vi "Main.vi"() -> ()   [LabVIEW 2013]
doc: "This template is for the Queued Message Handler design pattern.\n\nThe Event Handling Loop generates messages based on user interface actions.\n\nThe Message Handling Loop processes messages generated by the Event Handling Loop, or by other messages. The messages are string values, so new messages can be added easily to the Message Cases case structure in the Message Handling Loop. Each message cluster can also provide an optional value for Message Data, which is a variant that can be converted to whatever message-specific data is required."
uses:
  controls/UI Data.ctl
  Message Queue/Message Queue.lvlib
  User Event - Stop/User Event - Stop.lvlib
  <vilib>/vision/Image Controls.llb/IMAQ Image.ctl
  FPGA/FPGA Frame Grabbing.lvlib
  <vilib>/vision/NI_Vision_Development_Module.lvlib
  Image Processing/Image Processing.lvlib
  Common/State Machines/State Machine Lib.lvlib
  Message Passing/Main MsgQ.lvlib
  Message Passing/MsgQ Loops enum.ctl
  Sectors/Number of Wing Sector.ctl
panel:
  in  "Start Serial Server":bool=TRUE
  out "Wingbeat Amplitude Graph":dynamicdata(graph)
  in  "Stop Charts":bool
  in  "NumWingSectors":T1=12 items=["1"=1, "2"=2, "4"=4, "8"=8, "16"=16]
  in  "Wing ROIs":T2
  out "combo mask":T3(plugin-control)
  out "right \nannulus":T4={"Center X"=1090, "Center Y"=659, "Inner Radius"=200, "Outer Radius"=405, "Start Angle"=0.0, "End Angle"=90.0} {"End Angle" format="%.2f"; "Start Angle" format="%.2f"; "Center X" scale=0.0..1024.0}
  out "right masked image":T3(plugin-control)
  out "right mask":T3(plugin-control)
  out "left annulus":T4={"Center X"=929, "Center Y"=663, "Inner Radius"=200, "Outer Radius"=405, "Start Angle"=90.0, "End Angle"=180.0} {"End Angle" format="%.2f"; "Start Angle" format="%.2f"; "Center X" scale=0.0..1024.0}
  out "left masked image":T3(plugin-control)
  out "left mask":T3(plugin-control)
  in  "Accept Threshold":bool
  in  "Threshold Range":cluster{"Lower value":dbl, "Upper value":dbl}={"Lower value"=106.82432432432432, "Upper value"=255.0} {"Upper value" min=0.0 max=255.0 scale=0.0..255.0; "Lower value" min=0.0 max=255.0 scale=0.0..255.0}
  out "FPGA image info":T7={"Image Type"=0, "Unit"=enum."Undefined", "X Resolution"=2040, "Y Resolution"=1088, "X Step"=1.0, "Y Step"=1.0, "Image Name"="Image"} {"Image Type" items=["Grayscale (U8)", "Grayscale (I16)", "Grayscale (SGL)", "Complex (CSG)", "RGB (U32)", "HSL (U32)", "RGB (U64)", "Grayscale (U16)"]}
  out "Processed Image":T3(plugin-control)
  in  "Stream?":bool
  out "FPGA Image":T3(plugin-control)
  in  "Save Mask Coordinates":bool
  in  "Test Visual Response":bool
  in  "Test FPGA":bool
  out "Status Update":string="VI Stopped"
  in  "Define Mask":bool
  in  "Acquire Image":bool
  in  "Stop":bool
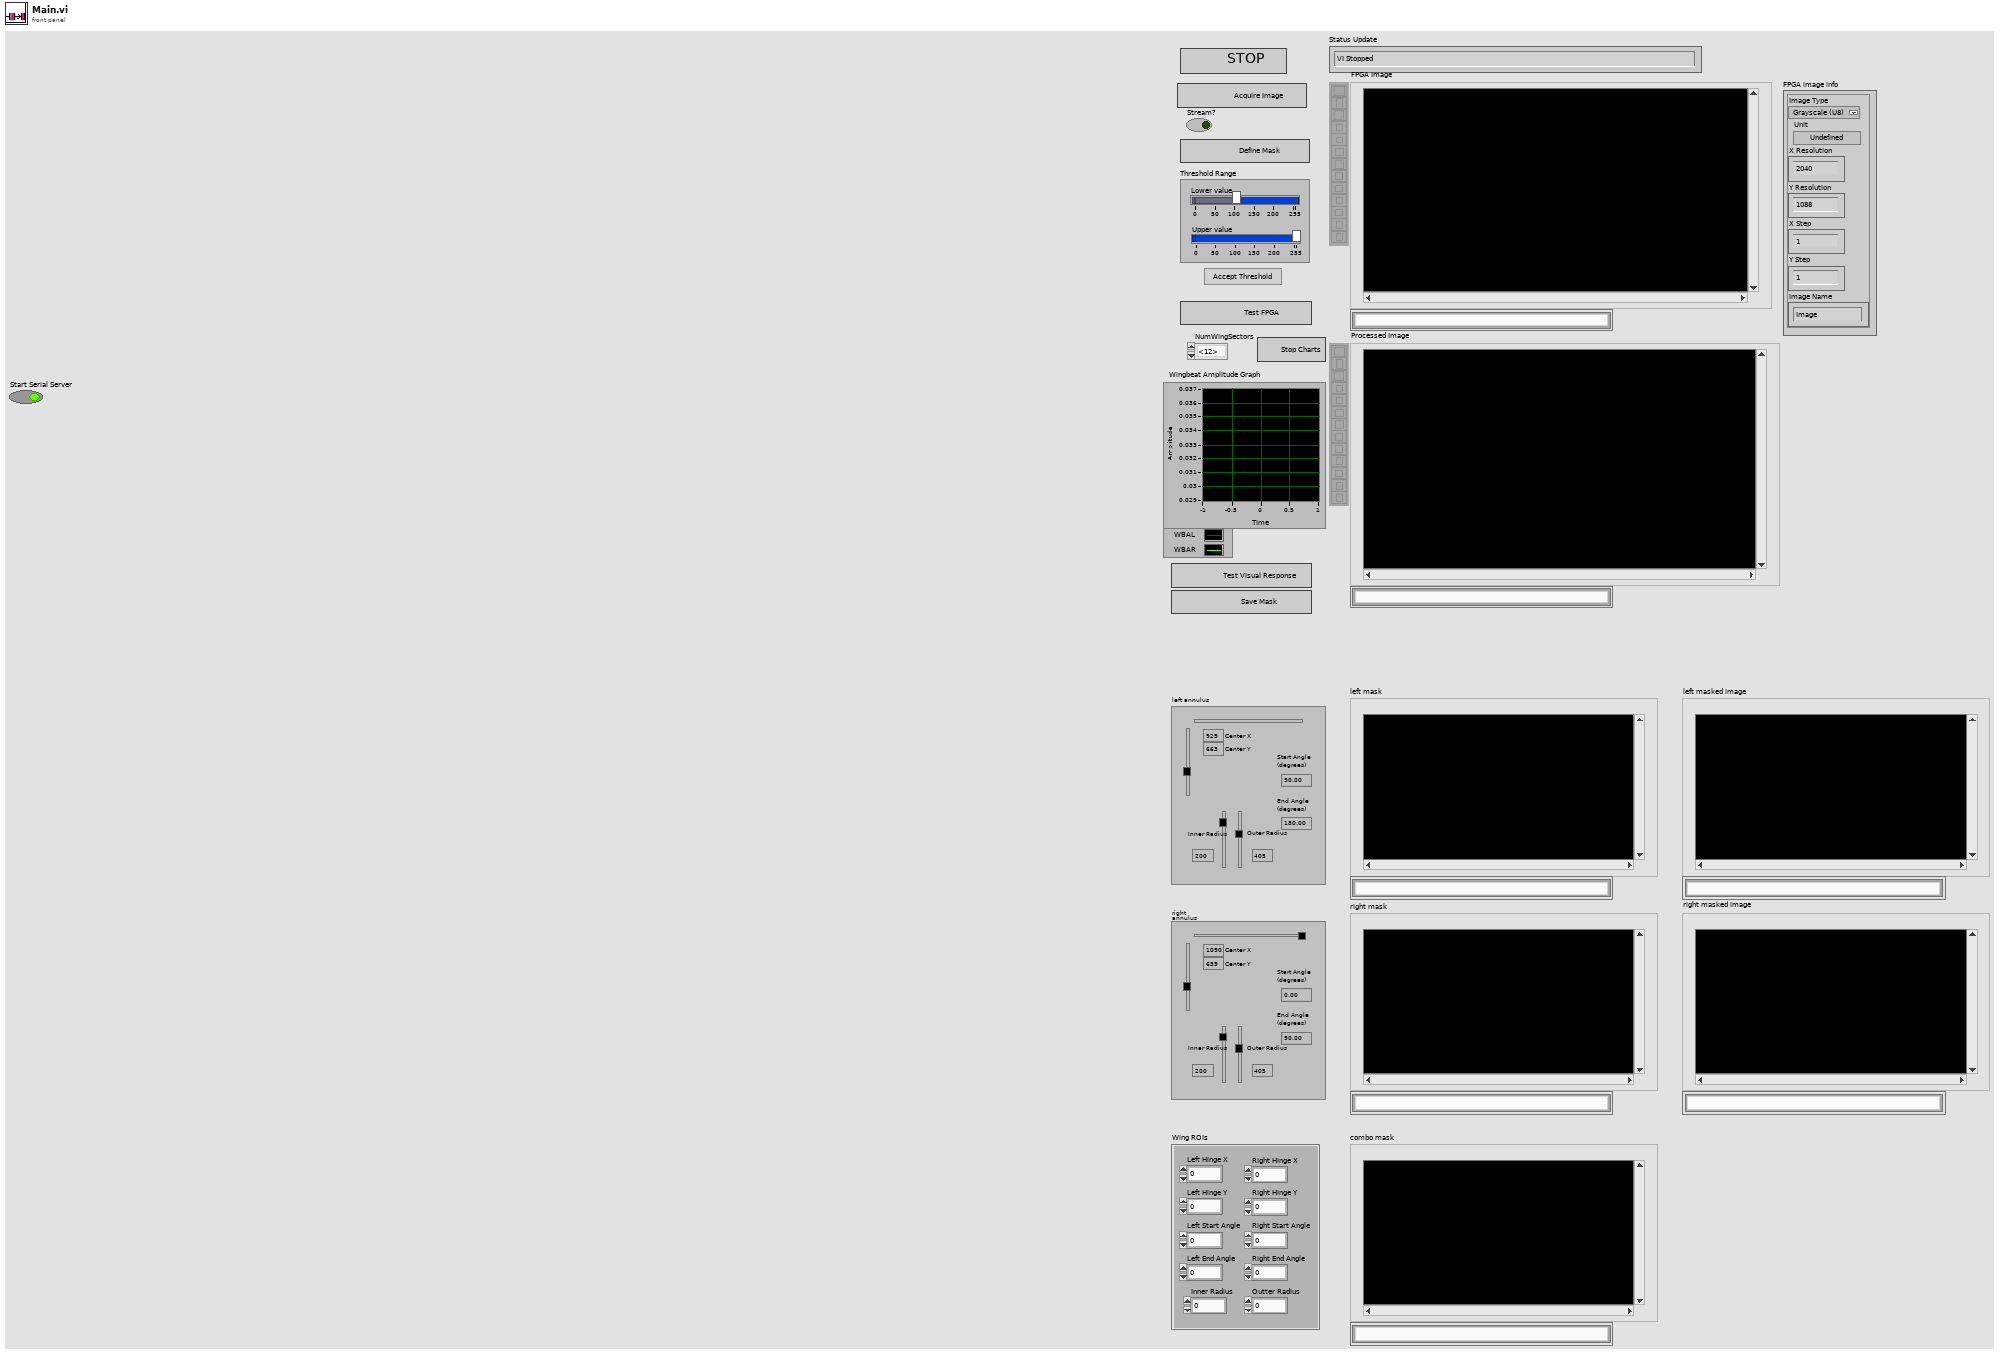
[diagram p1: front panel]
types:
  T1 = typedef "Number of Wing Sector.ctl" = u8
  T2 = cluster{"Left Hinge X":u16, "Left Hinge Y":u16, "Inner Radius":u16, "Outter Radius":u16, "Right Hinge X":u16, "Right Hinge Y":u16, "Right Start Angle":i16, "Right End Angle":i16, "Left Start Angle":i16, "Left End Angle":i16}
  T3 = typedef "IMAQ Image.ctl" = refnum<image>
  T4 = typedef "IMAQ Circle" = cluster{"Center X":i32, "Center Y":i32, "Inner Radius":i32, "Outer Radius":i32, "Start Angle":dbl, "End Angle":dbl}
  T5 = typedef "Image Type" = u32
  T6 = typedef "Image Unit" = enum32{"Undefined", "Angström", "Micrometer", "Millimeter", "Centimeter", "Meter", "Kilometer", "Microinch", "Inch", "Feet", "Nautical miles", "Standard miles", "Steps"}
  T7 = cluster{"Image Type":T5, "Unit":T6, "X Resolution":i32, "Y Resolution":i32, "X Step":sgl, "Y Step":sgl, "Image Name":string}
  T8 = typedef "UI Data.ctl" = cluster{"Boolean <Replace Me>":bool, "Initial Message":string, "Numeric <Replace Me>":dbl, "Acquire Image Ref":refnum<vi>, "Define Mask Ref":refnum<vi>, "Status Update Ref":refnum<vi>, "Stop Button Ref":refnum<vi>, "FPGA Image":T3, "Processed Image":T3, "Left Annulus":cluster{"Center X":i32, "Center Y":i32, "Inner Radius":i32, "Outer Radius":i32, "Start Angle":dbl, "End Angle":dbl}, "Right Annulus":cluster{"Center X":i32, "Center Y":i32, "Inner Radius":i32, "Outer Radius":i32, "Start Angle":dbl, "End Angle":dbl}}
  T9 = typedef "State Machine Lib.lvlib/STATE cluster.ctl" = cluster{"State":string, "Parameters":variant}
  T10 = typedef "Main MsgQ.lvlib/MsgQ Loops enum.ctl" = enum16{"User Interface", "Image Acq"}
  T11 = typedef "Message Queue.lvlib/All Message Queues.ctl" = cluster{"UI":refnum<queue>}
  T12 = cluster{"Center X":i32, "Center Y":i32, "Inner Radius":i32, "Outer Radius":i32, "Start Angle":dbl, "End Angle":dbl}
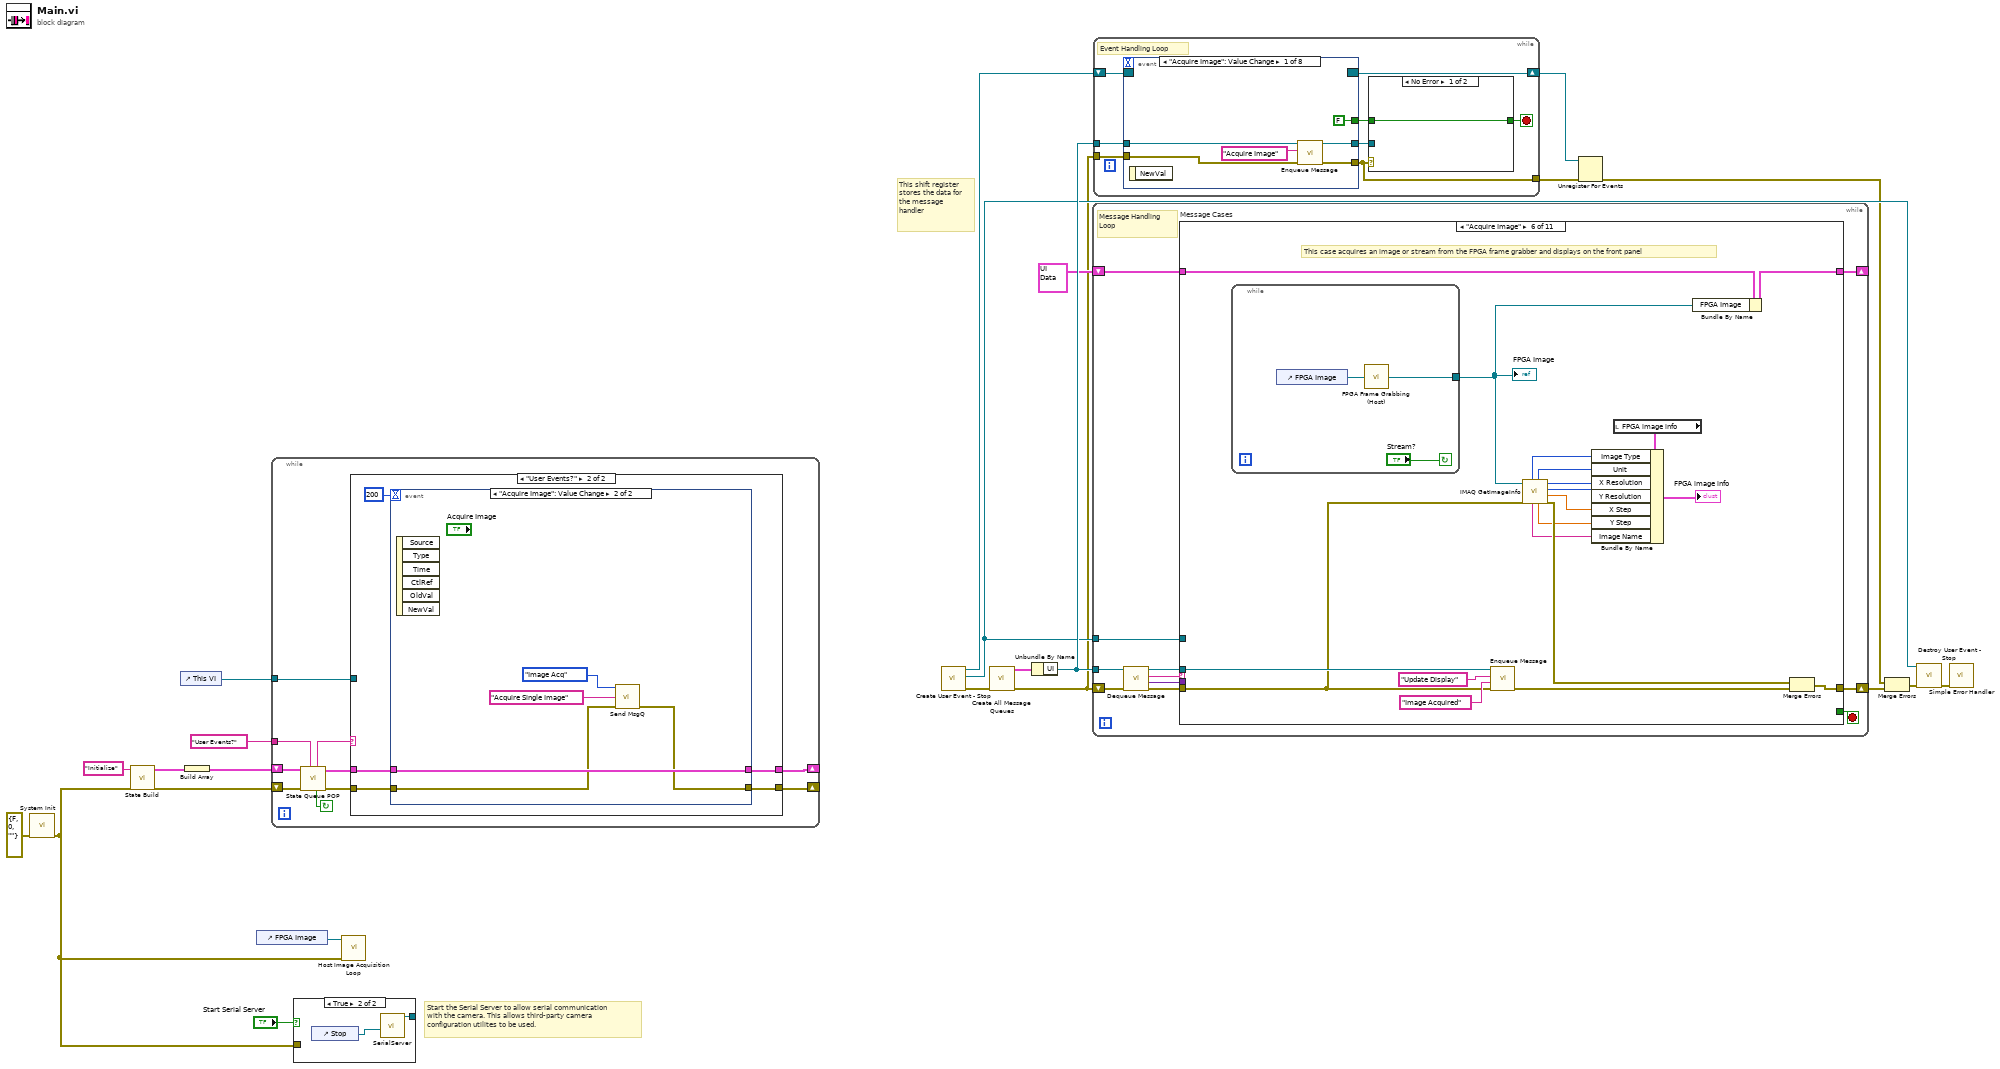
[diagram p0: block diagram]
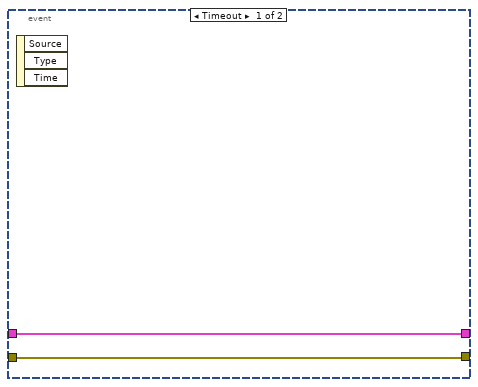
[diagram p3: hidden frame]
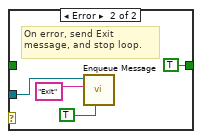
[diagram p5: hidden frame]
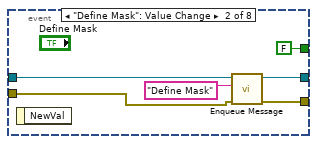
[diagram p6: hidden frame]
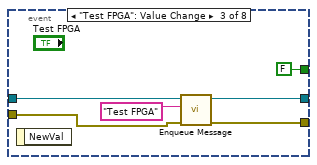
[diagram p7: hidden frame]
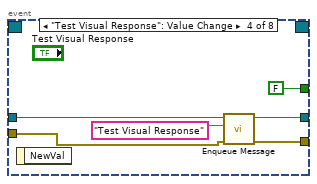
[diagram p8: hidden frame]
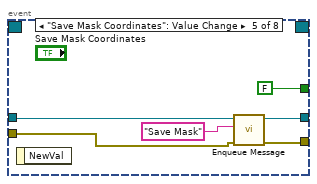
[diagram p9: hidden frame]
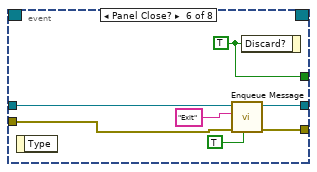
[diagram p10: hidden frame]
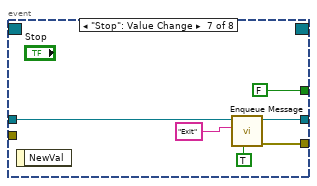
[diagram p11: hidden frame]
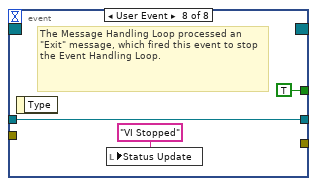
[diagram p12: hidden frame]
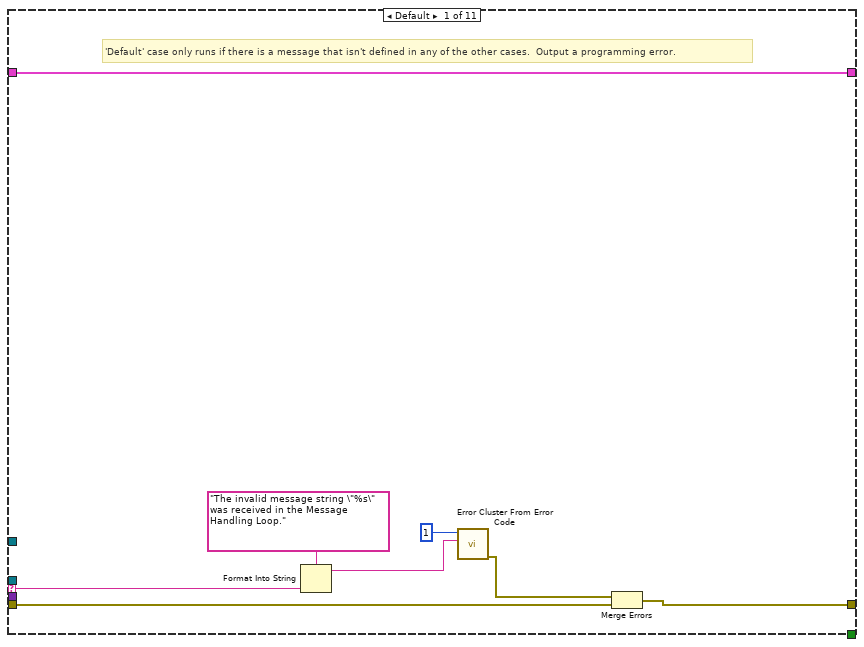
[diagram p13: hidden frame]
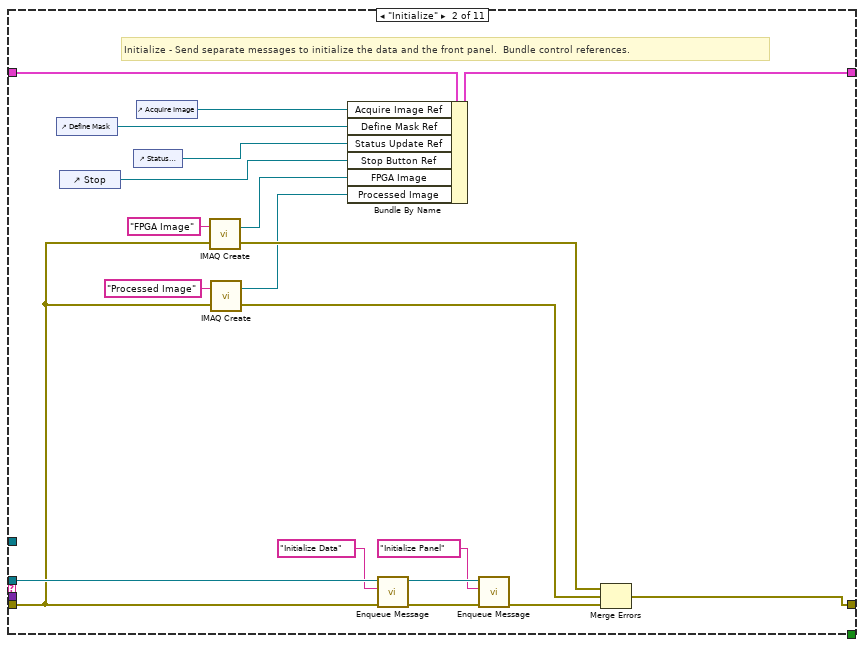
[diagram p14: hidden frame]
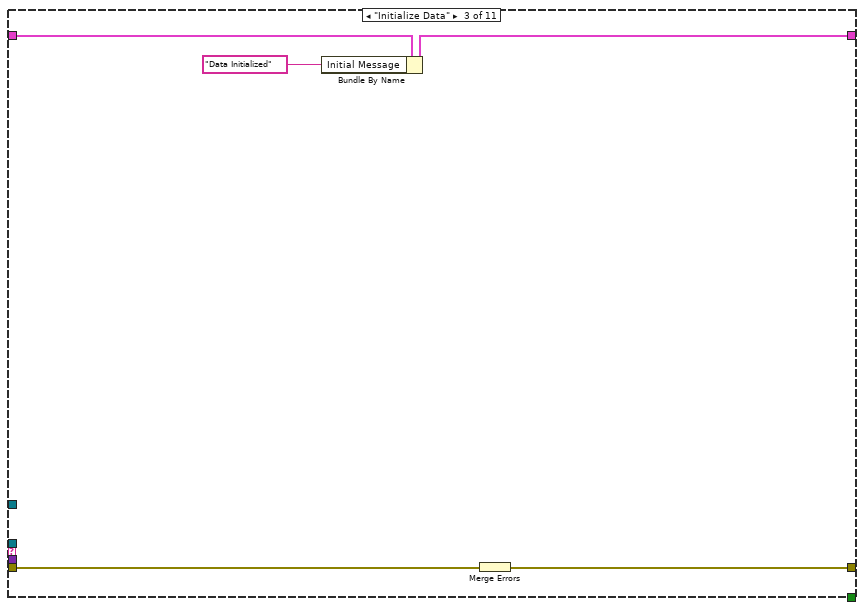
[diagram p15: hidden frame]
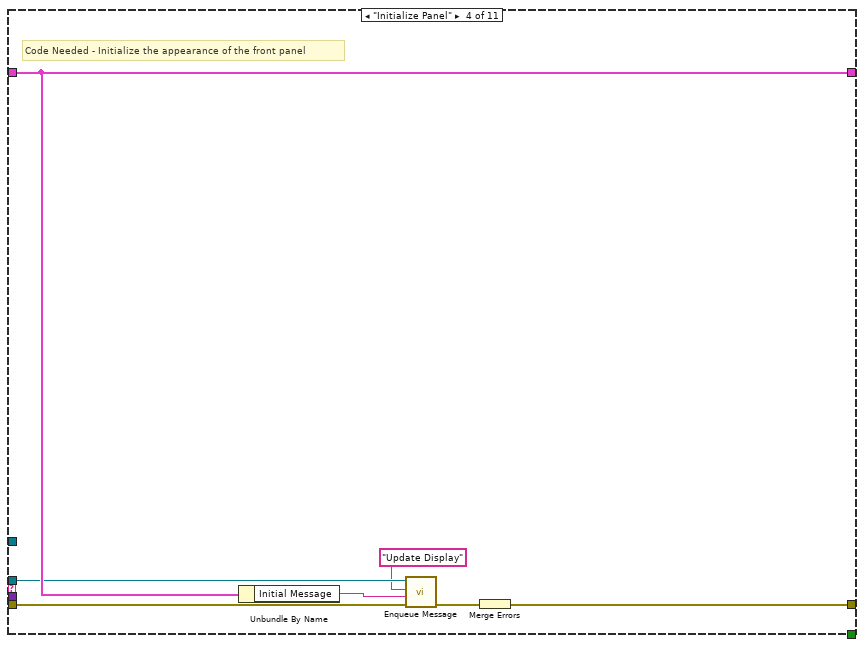
[diagram p16: hidden frame]
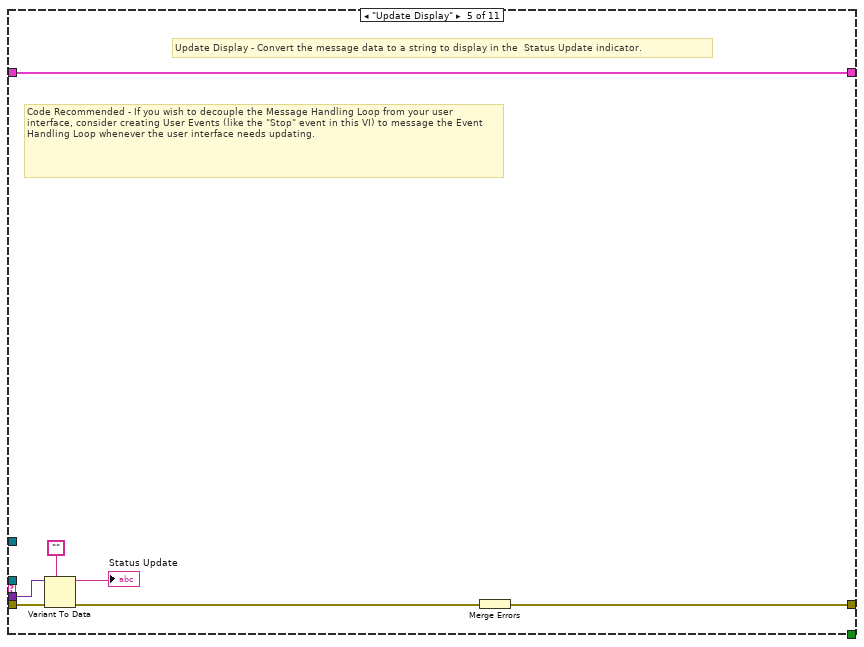
[diagram p17: hidden frame]
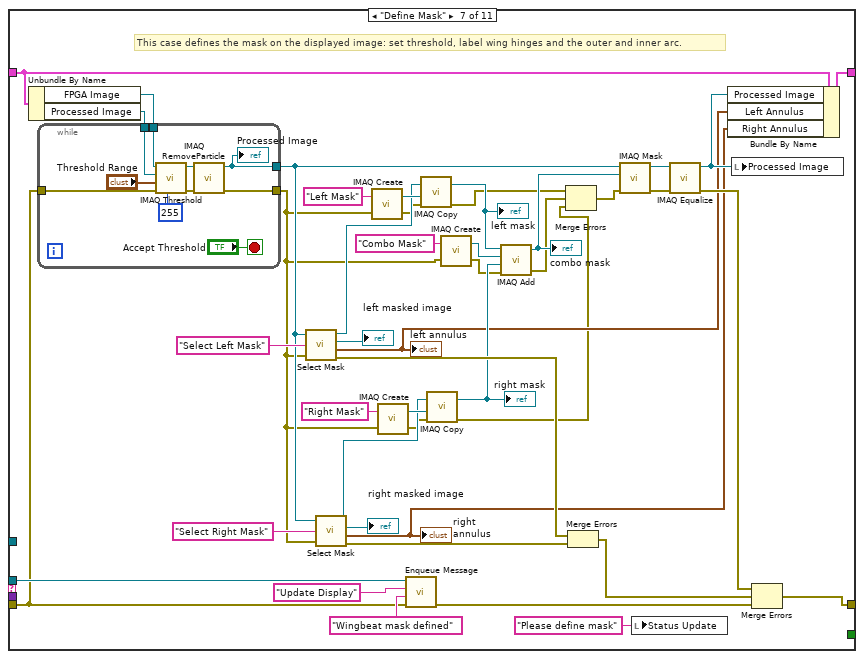
[diagram p18: hidden frame]
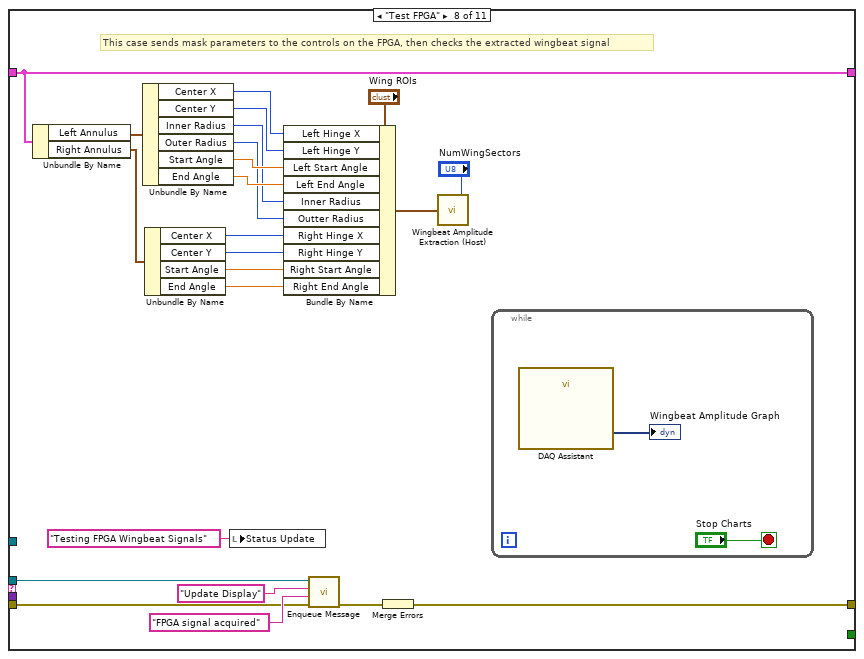
[diagram p19: hidden frame]
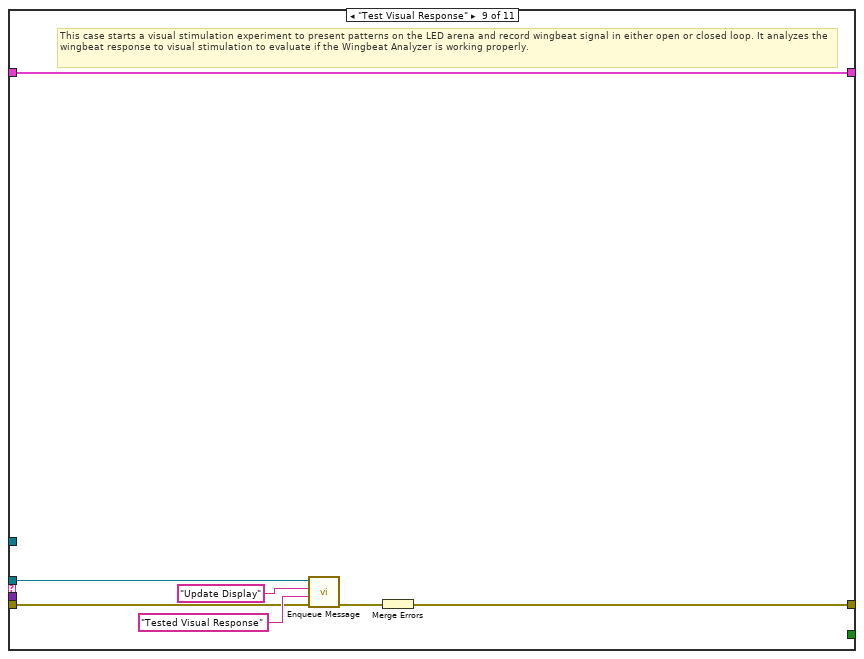
[diagram p20: hidden frame]
diagram:
  # "Start the Serial Server to allow serial communication\nwith the camera. This allows third-party camera\nconfiguration utilites to be used."
  # "This shift register\nstores the data for the message handler"
  n1 = call "System Init.vi"("error in (no error)"=errorcluster {"status"=FALSE, "code"=0, "source"=""}) -> ("error out"=w7:errorcluster)  [unwired: 10 in]
  n2 = call "State Build.vi"("error in (no error)"=w7, "State"="Initialize") -> ("error out"=w3:errorcluster, "State Out"=w5:T9)  [unwired: 8 in]
  n3 = control-ref of="This VI"() -> (w1:refnum<vi>)
  n4 = Build Array(w5) -> (w4:T9[])
  n5 = control-ref of="FPGA Image"() -> (w10:refnum<vi>)
  n6 = while {
    shift-right: [w27] -> _
    shift-left: w4 -> [w33]
    shift-right: [w25] -> _
    shift-left: w3 -> [w32]
    tunnel: "User Events?" ("State") -> [w30]
    tunnel: w1 -> [w28]
    stop <- w31 continue-if-true
    n7 = call "State Queue POP.vi"("Default state"=w30, "error in (no error)"=w32, "State que in"=w33) -> ("error out"=w24:errorcluster, "State que out"=w26:T9[], "Not Exit?"=w31:bool, "State case out"=w29:string)  [unwired: 4 in, 1 out]
    n8 = case shown="\"User Events?\"" w29 {
      tunnel: w28 -> [_ _]
      tunnel: [_ w37] -> w27
      tunnel: w26 -> [_ w36]
      tunnel: [_ w35] -> w25
      tunnel: w24 -> [_ w34]
      frame "False", Default {
      }
      frame "User Events?" {
        n9 = event shown="[1] \"Acquire Image\": Value Change" {
          selector: _ -> [_ _]
          dyn-events: _ -> [_ _]
          timeout: 200 -> [_ _]
          tunnel: [w40 w44] -> w37
          tunnel: w36 -> [w40 w44]
          tunnel: [w39 w41] -> w35
          tunnel: w34 -> [w39 w42]
          event Timeout {
            n10 = event-data() -> ()  [unwired: 1 in, 3 out]
          }
          event "Acquire Image": Value Change {
            n11 = event-data() -> ()  [unwired: 1 in, 6 out]
            n12 = call "Send MsgQ.vi"("error in (no error)"=w42, "Message String"="Acquire Single Image", "Send to MsgQ"=MsgQ_Loops_enum."Image Acq") -> ("error out"=w41:errorcluster)  [unwired: 8 in]
          }
        }
      }
    }
  }
  n13 = case shown="True" "Start Serial Server" {
    tunnel: [_ w47] -> _
    tunnel: w7 -> [_ _]
    frame False {
    }
    frame True {
      n14 = control-ref of="Stop"() -> (w46:refnum<vi>)
      n15 = call "SerialServer.vi"("Stop Refnum"=w46) -> ("FPGA VI Reference Out"=w47:refnum<k20>)  [unwired: 6 in]
    }
  }
  n16 = call "Host Image Acquisition Loop.vi"("error in"=w7, "Image Reference"=w10) -> ()  [unwired: 9 in, 1 out]
  n17 = call "Create User Event - Stop.vi"() -> ("error out"=w19:errorcluster, "User Event - Stop"=w16:refnum<user-event>, "Stop Event Registration Refnum"=w20:refnum<event-registration>)  [unwired: 9 in]
  n18 = call "Create All Message Queues.vi"("error in (no error)"=w19) -> ("error out"=w11:errorcluster, "Message Queues out"=w23:T11)  [unwired: 9 in]
  n19 = Unbundle By Name(w23) -> ("UI"=w21:refnum<queue>)
  n20 = while {
    tunnel: w21 -> [w48]
    shift-right: [w57] -> _
    shift-left: T8 {"Boolean <Replace Me>"=TRUE, "Initial Message"="", "Numeric <Replace Me>"=0.0, "Acquire Image Ref"=refnum, "Define Mask Ref"=refnum, "Status Update Ref"=refnum, "Stop Button Ref"=refnum, "FPGA Image"=refnum, "Processed Image"=refnum, "Left Annulus"={"Center X"=0, "Center Y"=0, "Inner Radius"=0, "Outer Radius"=0, "Start Angle"=0.0, "End Angle"=0.0}, "Right Annulus"={"Center X"=0, "Center Y"=0, "Inner Radius"=0, "Outer Radius"=0, "Start Angle"=0.0, "End Angle"=0.0}} ("Data Cluster") -> [w58]
    tunnel: w16 -> [w54]
    shift-right: [w55] -> w22
    shift-left: w11 -> [w53]
    stop <- w56 stop-if-true
    # "Message Handling Loop"
    n21 = call "Dequeue Message.vi"("error in (no error)"=w53, "Message Queue"=w48) -> ("error out"=w52:errorcluster, "Message Data"=w50:variant, "Message"=w51:string, "dup Message Queue"=w49:refnum<queue>)  [unwired: 6 in]
    n22 = case "Message Cases" shown="\"Acquire Image\"" w51 {
      selector: w51 -> [w64 _ _ _ _ _ _ _ _ _ _]
      tunnel: w49 -> [_ w84 _ w95 _ w122 w171 w200 w208 w216 w232]
      tunnel: w52 -> [w61 w69 w91 w96 w103 w117 w168 w201 w209 w214 w221]
      tunnel: [w59 w71 w87 w97 w104 w124 w128 w199 w207 w219 w228] -> w55
      tunnel: w58 -> [w66 w81 w90 w98 w105 w119 w167 w198 w213 w220 w231]
      tunnel: [w66 w80 w89 w98 w105 w118 w166 w198 w213 w220 w231] -> w57
      tunnel: [_ _ _ _ _ _ _ _ _ _ TRUE] -> w56
      tunnel: w50 -> [_ _ _ _ w102 _ _ _ _ _ _]
      tunnel: w54 -> [_ _ _ _ _ _ _ _ _ _ w227]
      frame Default {
        # "'Default' case only runs if there is a message that isn't defined in any of the other cases.  Output a programming error."
        n23 = Format Into String(format string="The invalid message string \"%s\" was received in the Message Handling Loop." ("Unknown Message Error Text"), w64) -> (resulting string=w62:string)  [unwired: 2 in, 1 out]
        n24 = call <vilib>:"Error Cluster From Error Code.vi"("error message (\"\")"=w62, "error code (0)"=1) -> ("error out"=w60:errorcluster)  [unwired: 7 in]
        n25 = Merge Errors(w60, w61) -> (w59:errorcluster)
      }
      frame "Initialize" {
        # "Initialize - Send separate messages to initialize the data and the front panel.  Bundle control references."
        n26 = control-ref of="Define Mask"() -> (w78:refnum<vi>)
        n27 = control-ref of="Stop"() -> (w76:refnum<vi>)
        n28 = control-ref of="Status Update"() -> (w77:refnum<vi>)
        n29 = control-ref of="Acquire Image"() -> (w79:refnum<vi>)
        n30 = call "IMAQ Create"("Image Name"="FPGA Image", "error in (no error)"=w69) -> ("New Image"=w74:T3, "error out"=w70:errorcluster)  [unwired: 3 in]
        n31 = call "IMAQ Create"("Image Name"="Processed Image", "error in (no error)"=w69) -> ("New Image"=w67:T3, "error out"=w68:errorcluster)  [unwired: 3 in]
        n32 = Bundle By Name(cluster=w81, "Acquire Image Ref"=w79, "Define Mask Ref"=w78, "Status Update Ref"=w77, "Stop Button Ref"=w76, "FPGA Image"=w74, "Processed Image"=w67) -> (w80:T8)
        n33 = call "Enqueue Message.vi"("error in (no error)"=w69, "Message"="Initialize Data", "Message Queue"=w84) -> ("error out"=w86:errorcluster, "dup Message Queue"=w85:refnum<queue>)  [unwired: 7 in]
        n34 = call "Enqueue Message.vi"("error in (no error)"=w86, "Message"="Initialize Panel", "Message Queue"=w85) -> ("error out"=w72:errorcluster)  [unwired: 7 in, 1 out]
        n35 = Merge Errors(w70, w68, w72) -> (w71:errorcluster)
      }
      frame "Initialize Data" {
        n36 = Bundle By Name(cluster=w90, "Initial Message"="Data Initialized") -> (w89:T8)
        n37 = Merge Errors(w91) -> (w87:errorcluster)
      }
      frame "Initialize Panel" {
        # "Code Needed - Initialize the appearance of the front panel"
        n38 = Unbundle By Name(w98) -> ("Initial Message"=w92:string)
        n39 = call "Enqueue Message.vi"("error in (no error)"=w96, "Message Data"=w92, "Message"="Update Display", "Message Queue"=w95) -> ("error out"=w94:errorcluster)  [unwired: 6 in, 1 out]
        n40 = Merge Errors(w94) -> (w97:errorcluster)
      }
      frame "Update Display" {
        # "Code Recommended - If you wish to decouple the Message Handling Loop from your user interface, consider creating User Events (like the \"Stop\" event in this VI) to message the Event Handling Loop whenever the user interface needs updating."
        # "Update Display - Convert the message data to a string to display in the  Status Update indicator."
        n41 = Variant To Data(error in=w103, type="", Variant=w102) -> (data=→"Status Update":string, error out=w100:errorcluster)
        n42 = Merge Errors(w100) -> (w104:errorcluster)
      }
      frame "Acquire Image" {
        # "This case acquires an image or stream from the FPGA frame grabber and displays on the front panel"
        n43 = while {
          tunnel: [w126] -> w106
          stop <- "Stream?" continue-if-true
          n44 = control-ref of="FPGA Image"() -> (w125:refnum<vi>)
          n45 = call "FPGA Frame Grabbing (Host).vi"("Ctl Refnum"=w125) -> ("Image"=w126:T3)
        }
        "FPGA Image" <- w106
        n46 = call "Enqueue Message.vi"("error in (no error)"=w117, "Message Data"="Image Acquired" ("\"Do Something\" button pressed"), "Message"="Update Display", "Message Queue"=w122) -> ("error out"=w123:errorcluster)  [unwired: 6 in, 1 out]
        n47 = call "IMAQ GetImageInfo"("error in (no error)"=w117, "Image"=w106) -> ("error out"=w116:errorcluster, "X Step"=w111:sgl, "Y Resolution"=w112:i32, "X Resolution"=w113:i32, "Y Step"=w110:sgl, "Unit"=w114:T6, "Image Name"=w109:string, "Image Type"=w115:T5)  [unwired: 2 in]
        n48 = local read "FPGA image info"() -> (w107:T7)
        n49 = Bundle By Name(cluster=w107, "Image Type"=w115, "Unit"=w114, "X Resolution"=w113, "Y Resolution"=w112, "X Step"=w111, "Y Step"=w110, "Image Name"=w109) -> (→"FPGA image info":T7)
        n50 = Bundle By Name(cluster=w119, "FPGA Image"=w106) -> (w118:T8)
        n51 = Merge Errors(w116, w123) -> (w124:errorcluster)
      }
      frame "Define Mask" {
        # "This case defines the mask on the displayed image: set threshold, label wing hinges and the outer and inner arc."
        n52 = Unbundle By Name(w167) -> ("FPGA Image"=w165:T3, "Processed Image"=w164:T3)
        n53 = while {
          tunnel: w168 -> [w181]
          tunnel: w165 -> [w180]
          tunnel: w164 -> [w179]
          tunnel: [w172] -> w150
          tunnel: [w174] -> w134
          stop <- "Accept Threshold" stop-if-true
          n54 = call "IMAQ Threshold"("Replace Value"=u8 255, "error in (no error)"=w181, "Range"="Threshold Range", "Image Dst"=w179, "Image Src"=w180) -> ("error out"=w177:errorcluster, "Image Dst Out"=w176:T3)  [unwired: 1 in, 4 out]
          n55 = call "IMAQ RemoveParticle"("error in (no error)"=w177, "Image Src"=w176) -> ("error out"=w174:errorcluster, "Image Dst Out"=w172:T3)  [unwired: 5 in, 3 out]
          "Processed Image" <- w172
        }
        n56 = call "Select Mask.vi"("Read \nImage"=w150, "Prompt"="Select Left Mask", "error in"=w134) -> ("mask"=w143:T3, "Masked \nImage"=→"left masked image":T3, "Annulus"=w139:T4, "error out"=w154:errorcluster)  [unwired: 1 out]
        "left annulus" <- w139
        n57 = call "Select Mask.vi"("Read \nImage"=w150, "Prompt"="Select Right Mask", "error in"=w134) -> ("mask"=w141:T3, "Masked \nImage"=→"right masked image":T3, "Annulus"=w138:T4, "error out"=w153:errorcluster)  [unwired: 1 out]
        "right \nannulus" <- w138
        n58 = call "IMAQ Create"("Image Name"="Left Mask", "error in (no error)"=w134) -> ("New Image"=w146:T3, "error out"=w137:errorcluster)  [unwired: 3 in]
        n59 = call "IMAQ Create"("Image Name"="Right Mask", "error in (no error)"=w134) -> ("New Image"=w144:T3, "error out"=w136:errorcluster)  [unwired: 3 in]
        n60 = call "Enqueue Message.vi"("error in (no error)"=w168, "Message Data"="Wingbeat mask defined" ("\"Do Something Else\" button pressed"), "Message"="Update Display", "Message Queue"=w171) -> ("error out"=w129:errorcluster)  [unwired: 6 in, 1 out]
        n61 = call "IMAQ Copy"("error in (no error)"=w137, "Image Dst"=w146, "Image Src"=w143) -> ("error out"=w133:errorcluster, "Image Dst Out"=w142:T3)  [unwired: 3 in]
        "left mask" <- w142
        n62 = call "IMAQ Copy"("error in (no error)"=w136, "Image Dst"=w144, "Image Src"=w141) -> ("error out"=w131:errorcluster, "Image Dst Out"=w140:T3)  [unwired: 3 in]
        "right mask" <- w140
        n63 = call "IMAQ Create"("Image Name"="Combo Mask", "error in (no error)"=w134) -> ("New Image"=w151:T3, "error out"=w135:errorcluster)  [unwired: 3 in]
        n64 = call "IMAQ Add"("Image Src A"=w142, "Image Dst"=w151, "Image Src B"=w140, "error in (no error)"=w135) -> ("Image Dst Out"=w148:T3, "error out"=w132:errorcluster)  [unwired: 3 in]
        "combo mask" <- w148
        n65 = Merge Errors(w133, w132, w131) -> (w130:errorcluster)
        n66 = Merge Errors(w154, w153) -> (w149:errorcluster)
        n67 = call "IMAQ Mask"("error in (no error)"=w130, "Image Mask"=w148, "Image Src"=w150) -> ("error out"=w159:errorcluster, "Image Dst Out"=w160:T3)  [unwired: 1 in, 1 out]
        n68 = local write "Status Update"("Please define mask" ("Status Update")) -> ()
        n69 = call "IMAQ Equalize"("error in (no error)"=w159, "Image Src"=w160) -> ("error out"=w162:errorcluster, "Image Dst Out"=w158:T3)  [unwired: 4 in, 4 out]
        n70 = Bundle By Name(cluster=w167, "Processed Image"=w158, "Left Annulus"=w139, "Right Annulus"=w138) -> (w166:T8)
        n71 = local write "Processed Image"(w158) -> ()
        n72 = Merge Errors(w162, w149, w129) -> (w128:errorcluster)
      }
      frame "Test FPGA" {
        # "This case sends mask parameters to the controls on the FPGA, then checks the extracted wingbeat signal"
        n73 = Unbundle By Name(w198) -> ("Left Annulus"=w197:T12, "Right Annulus"=w196:T12)
        n74 = Unbundle By Name(w197) -> ("Center X"=w194:i32, "Center Y"=w193:i32, "Inner Radius"=w190:i32, "Outer Radius"=w189:i32, "Start Angle"=w192:dbl, "End Angle"=w191:dbl)
        n75 = Unbundle By Name(w196) -> ("Center X"=w188:i32, "Center Y"=w187:i32, "Start Angle"=w186:dbl, "End Angle"=w185:dbl)
        n76 = local write "Status Update"("Testing FPGA Wingbeat Signals" ("Status Update")) -> ()
        n77 = Bundle By Name(cluster="Wing ROIs", "Left Hinge X"=w194, "Left Hinge Y"=w193, "Left Start Angle"=w192, "Left End Angle"=w191, "Inner Radius"=w190, "Outter Radius"=w189, "Right Hinge X"=w188, "Right Hinge Y"=w187, "Right Start Angle"=w186, "Right End Angle"=w185) -> (w184:T2)
        n78 = call "Enqueue Message.vi"("error in (no error)"=w201, "Message Data"="FPGA signal acquired" ("\"Do Something\" button pressed"), "Message"="Update Display", "Message Queue"=w200) -> ("error out"=w204:errorcluster)  [unwired: 6 in, 1 out]
        n79 = Merge Errors(w204) -> (w199:errorcluster)
        n80 = call "Wingbeat Amplitude Extraction (Host).vi"("NumWingSectors"="NumWingSectors", "Wing ROIs"=w184) -> ()
        n81 = while {
          stop <- "Stop Charts" stop-if-true
          n82 = call "DAQ Assistant"() -> ("data"=→"Wingbeat Amplitude Graph":dynamicdata)  [unwired: 17 in, 2 out]
        }
      }
      frame "Test Visual Response" {
        # "This case starts a visual stimulation experiment to present patterns on the LED arena and record wingbeat signal in either open or closed loop. It analyzes the wingbeat response to visual stimulation to evaluate if the Wingbeat Analyzer is working properly."
        n83 = call "Enqueue Message.vi"("error in (no error)"=w209, "Message Data"="Tested Visual Response" ("\"Do Something\" button pressed"), "Message"="Update Display", "Message Queue"=w208) -> ("error out"=w212:errorcluster)  [unwired: 6 in, 1 out]
        n84 = Merge Errors(w212) -> (w207:errorcluster)
      }
      frame "Save Mask" {
        # "This case saves the current mask parameters to disk so other VIs can use them to control the FPGA"
        n85 = call "Enqueue Message.vi"("error in (no error)"=w214, "Message Data"="Mask parameters saved" ("\"Do Something Else\" button pressed"), "Message"="Update Display", "Message Queue"=w216) -> ("error out"=w215:errorcluster)  [unwired: 6 in, 1 out]
        n86 = Merge Errors(w215) -> (w219:errorcluster)
      }
      frame "Exit" {
        # "Stop the VI"
        # "Release the message queue reference"
        # "Code Needed - Add any required cleanup code here"
        n87 = call "Fire User Event - Stop.vi"("User Event - Stop"=w227) -> ("error out"=w226:errorcluster)  [unwired: 10 in]
        n88 = Release Queue(queue=w232, error in (no error)=w221) -> (error out=w229:errorcluster)  [unwired: 1 in, 2 out]
        n89 = call "IMAQ WindClose"("Close All Windows (False)"=TRUE, "error in (no error)"=w221) -> ("error out"=w223:errorcluster)  [unwired: 4 in]
        n90 = call "IMAQ Dispose"("All Images? (No)"=TRUE, "error in (no error)"=w223) -> ("error out"=w222:errorcluster)  [unwired: 4 in]
        n91 = Merge Errors(w222, w226, w229) -> (w228:errorcluster)
      }
    }
  }
  n92 = while {
    tunnel: w21 -> [w240]
    tunnel: [w236] -> w14
    shift-right: [w234] -> w13
    shift-left: w20 -> [w235]
    tunnel: w11 -> [w233]
    stop <- w238 stop-if-true
    # "Event Handling Loop"
    n93 = event shown="[0] \"Acquire Image\": Value Change" {
      selector: w235 -> [_ _ _ _ _ _ _ _]
      dyn-events: [_ _ _ _ _ _ _ _] -> w234
      timeout: _ -> [_ _ _ _ _ _ _ _]
      tunnel: [FALSE ("Discard?") FALSE ("Discard?") FALSE ("Discard?") FALSE ("Discard?") FALSE ("Discard?") w282 FALSE ("Discard?") TRUE ("Discard?")] -> w239
      tunnel: w240 -> [w251 w257 w263 w268 w273 w281 w288 w291]
      tunnel: [w250 w255 w260 w265 w270 w280 w287 _] -> w236
      tunnel: [w249 w256 w259 w267 w272 w279 w285 w291] -> w237
      tunnel: w233 -> [w247 w253 w261 w264 w271 w276 _ _]
      event "Acquire Image": Value Change {
        n94 = event-data() -> ()  [unwired: 1 in, 1 out]
        n95 = call "Enqueue Message.vi"("error in (no error)"=w247, "Message"="Acquire Image", "Message Queue"=w251) -> ("error out"=w250:errorcluster, "dup Message Queue"=w249:refnum<queue>)  [unwired: 7 in]
      }
      event "Define Mask": Value Change {
        n96 = event-data() -> ()  [unwired: 1 in, 1 out]
        n97 = call "Enqueue Message.vi"("error in (no error)"=w253, "Message"="Define Mask", "Message Queue"=w257) -> ("error out"=w255:errorcluster, "dup Message Queue"=w256:refnum<queue>)  [unwired: 7 in]
      }
      event "Test FPGA": Value Change {
        n98 = event-data() -> ()  [unwired: 1 in, 1 out]
        n99 = call "Enqueue Message.vi"("error in (no error)"=w261, "Message"="Test FPGA", "Message Queue"=w263) -> ("error out"=w260:errorcluster, "dup Message Queue"=w259:refnum<queue>)  [unwired: 7 in]
      }
      event "Test Visual Response": Value Change {
        n100 = event-data() -> ()  [unwired: 1 in, 1 out]
        n101 = call "Enqueue Message.vi"("error in (no error)"=w264, "Message"="Test Visual Response", "Message Queue"=w268) -> ("error out"=w265:errorcluster, "dup Message Queue"=w267:refnum<queue>)  [unwired: 7 in]
      }
      event "Save Mask Coordinates": Value Change {
        n102 = event-data() -> ()  [unwired: 1 in, 1 out]
        n103 = call "Enqueue Message.vi"("error in (no error)"=w271, "Message"="Save Mask", "Message Queue"=w273) -> ("error out"=w270:errorcluster, "dup Message Queue"=w272:refnum<queue>)  [unwired: 7 in]
      }
      event Panel Close? {
        w282 = TRUE ("Discard?")
        n104 = event-data() -> ()  [unwired: 1 in, 1 out]
        n105 = call "Enqueue Message.vi"("Priority Message? (F)"=TRUE, "error in (no error)"=w276, "Message"="Exit", "Message Queue"=w281) -> ("error out"=w280:errorcluster, "dup Message Queue"=w279:refnum<queue>)  [unwired: 6 in]
        n106 = event-data("Discard?"=w282) -> ()  [unwired: 1 in, 1 out]
      }
      event "Stop": Value Change {
        n107 = event-data() -> ()  [unwired: 1 in, 1 out]
        n108 = call "Enqueue Message.vi"("Priority Message? (F)"=TRUE, "Message"="Exit", "Message Queue"=w288) -> ("error out"=w287:errorcluster, "dup Message Queue"=w285:refnum<queue>)  [unwired: 7 in]
      }
      event User Event {
        # "The Message Handling Loop processed an \"Exit\" message, which fired this event to stop the Event Handling Loop."
        n109 = event-data() -> ()  [unwired: 1 in, 1 out]
        n110 = local write "Status Update"("VI Stopped" ("VI Stopped")) -> ()
      }
    }
    n111 = case shown="No Error" w236 {
      tunnel: [w241 TRUE ("Discard?")] -> w238
      tunnel: w239 -> [w241 _]
      tunnel: w237 -> [_ w244]
      frame No Error {
      }
      frame Error {
        # "On error, send Exit message, and stop loop."
        n112 = call "Enqueue Message.vi"("Priority Message? (F)"=TRUE, "Message"="Exit", "Message Queue"=w244) -> ()  [unwired: 7 in, 2 out]
      }
    }
  }
  n113 = Unregister For Events(event registration refnum=w13, error in=w14) -> (error out=w15:errorcluster)
  n114 = Merge Errors(w15, w22) -> (w17:errorcluster)
  n115 = call "Destroy User Event - Stop.vi"("error in (no error)"=w17, "User Event - Stop"=w16) -> ("error out"=w18:errorcluster)  [unwired: 9 in]
  n116 = call <vilib>:"Simple Error Handler.vi"("error in (no error)"=w18) -> ()  [unwired: 4 in, 5 out]
